vi "Stop Core.vi"(10 "final error code":i32 caption="最终错误代码", 11 "ParentActor in":refnum<class "ParentActor.lvclass"> caption="操作者输入") -> (3 "ParentActor out":refnum<class "ParentActor.lvclass"> caption="操作者输出")   [LabVIEW 2014, in "UnitTest.lvlib" / "ParentActor.lvclass"]
doc: "(<B>文件名</B>：Actor Framework.lvlib:Actor.lvclass:Stop Core.vi)\n\n定义停止前操作者的动作。使用<B>最终错误代码</B>输入判断操作者是否在出错时关闭。\n\n默认情况下，该方法不执行任何动作。子孙类重写该方法，定义出错时的操作，例如，关闭操作者核心方法初始的进程。"
uses:
  ParentActor.lvclass
  labview/1603/zsRobotSynergeticSystem/zsLib/zsActor/zsActor.lvclass
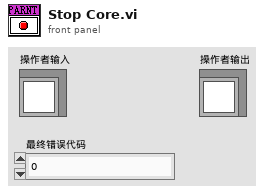
[diagram p1: front panel]
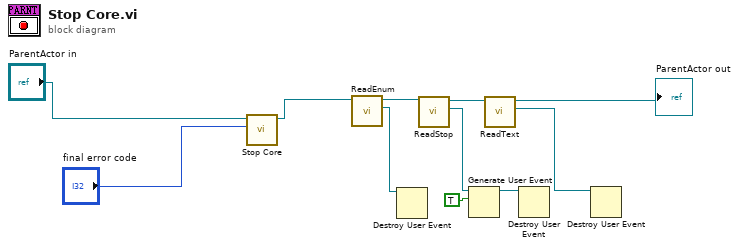
[diagram p0: block diagram]
diagram:
  n1 = call-parent "Stop Core.vi"("final error code"="final error code", "Actor in"="ParentActor in") -> ("Actor out"=w9:refnum<class "ParentActor.lvclass">)  [unwired: 9 in]
  n2 = call-dynamic "ReadEnum.vi"("zsActor输入"=w9) -> ("Enum"=w2:refnum<user-event>, "zsActor输出"=w8:refnum<class "ParentActor.lvclass">)  [unwired: 8 in, 1 out]
  n3 = Destroy User Event(user event=w2) -> ()  [unwired: 1 in, 1 out]
  n4 = call-dynamic "ReadStop.vi"("zsActor输入"=w8) -> ("Stop"=w4:refnum<user-event>, "zsActor输出"=w7:refnum<class "ParentActor.lvclass">)  [unwired: 8 in, 1 out]
  n5 = Generate User Event(user event=w4, event data cluster=TRUE ("event data")) -> (user event out=w5:refnum<user-event>)  [unwired: 2 in, 1 out]
  n6 = call-dynamic "ReadText.vi"("zsActor输入"=w7) -> ("Text"=w3:refnum<user-event>, "zsActor输出"=→"ParentActor out":refnum<class "ParentActor.lvclass">)  [unwired: 8 in, 1 out]
  n7 = Destroy User Event(user event=w5) -> ()  [unwired: 1 in, 1 out]
  n8 = Destroy User Event(user event=w3) -> ()  [unwired: 1 in, 1 out]
